vi "Periodic Tasks.vi"() -> ()   [LabVIEW 2011]
doc: "This VI runs in parallel to other tasks. It can contain as many user-defined periodic loops as you need. These can carry out PID or other sorts of timed response."
uses:
  Common/ADXL345 I2C Axis.ctl
  Robot Global Data.vi
panel:
  in  "Driving Sensor Enable":bool=TRUE
  out "Angle":dbl(knob) scale=0.0..360.0
  in  "Reset Zero Position":bool
  out "Robot Angle":dbl
  in  "Inertial Sensors Enable":bool=TRUE
  out "Direction":bool
  out "Voltage Turntable":dbl(knob) scale=160.0..230.0
  out "Acceleration X":dbl
  out "Acceleration Y":dbl
  out "Acceleration Z":dbl
  out "Voltage":dbl(knob) scale=90.0..140.0
  out "Average":dbl
  out "RPM 2":dbl
  out "RPM":dbl(knob) scale=0.0..4000.0
  out "Value":i32
  out "Sonar Distance":dbl
  in  "Shooting Sensor Enable":bool=TRUE
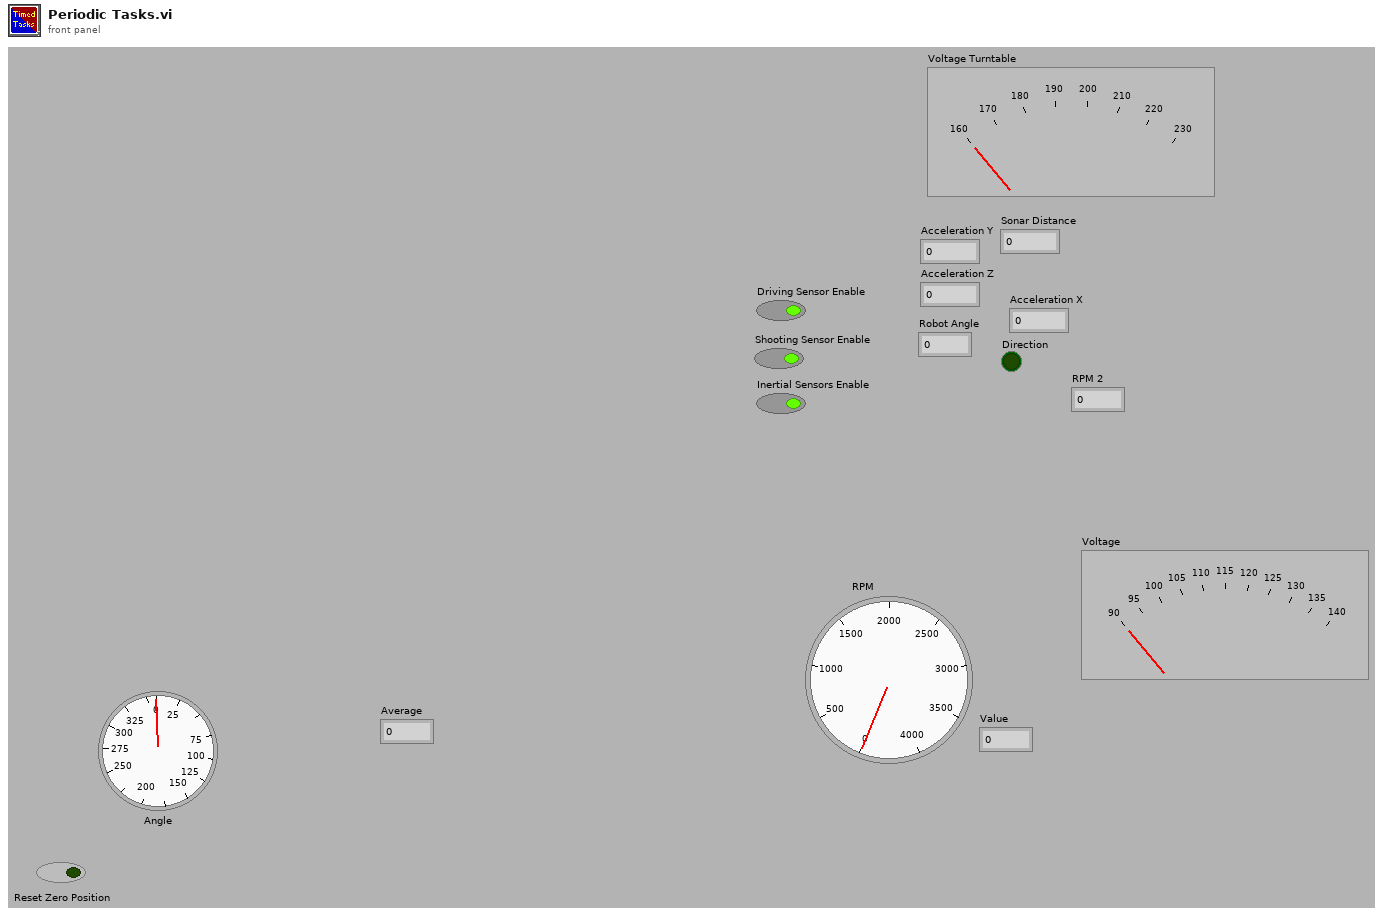
[diagram p1: front panel]
types:
  T1 = typedef "WPI_I2CDevRef.ctl" = cluster{"DevStatus":errorcluster, "Digital Module":T2, "Device Address":u8}
  T2 = typedef "FPGA_TypedefDigitalModule.ctl" = enum16{"Digital Module 1", "Digital Module 2"}
  T3 = typedef "WPI_AnalogChannelDevRef.ctl" = cluster{"DevStatus":errorcluster, "Analog Module":T4, "Analog Channel":T5}
  T4 = typedef "FPGA_TypedefAnalogModule.ctl" = enum16{"Analog Module 1", "Analog Module 2"}
  T5 = typedef "FPGA_AIChannel.ctl" = enum8{"AI 1", "AI 2", "AI 3", "AI 4", "AI 5", "AI 6", "AI 7", "AI 8", "Invalid"}
  T6 = typedef "WPI_CounterDevRef.ctl" = cluster{"DevStatus":errorcluster, "CntIndex":T7}
  T7 = typedef "FPGA_CounterCtrSystemIndex.ctl" = enum8{"Ctr 0", "Ctr 1", "Ctr 2", "Ctr 3", "Ctr 4", "Ctr 5", "Ctr 6", "Ctr 7", "Invalid"}
  T8 = typedef "WPI_GyroDevRef.ctl" = cluster{"DevStatus":errorcluster, "Analog Module":T4, "Analog Channel":T5, "Offset":dbl, "Gain (VoltsPerDegree/Second)":dbl}
  T9 = typedef "WPI_EncoderDevRef.ctl" = cluster{"DevStatus":errorcluster, "EncoderIndex":T10, "CounterIndex":T7, "DistancePerCount":dbl, "Decoding Type":T11}
  T10 = typedef "FPGA_EncoderIdx.ctl" = enum8{"Enc 0", "Enc 1", "Enc 2", "Enc 3", "Invalid"}
  T11 = typedef "WPI_EncoderType.ctl" = enum16{"1x", "2x", "4x"}
  T12 = typedef "ADXL345 I2C Axis.ctl" = u8
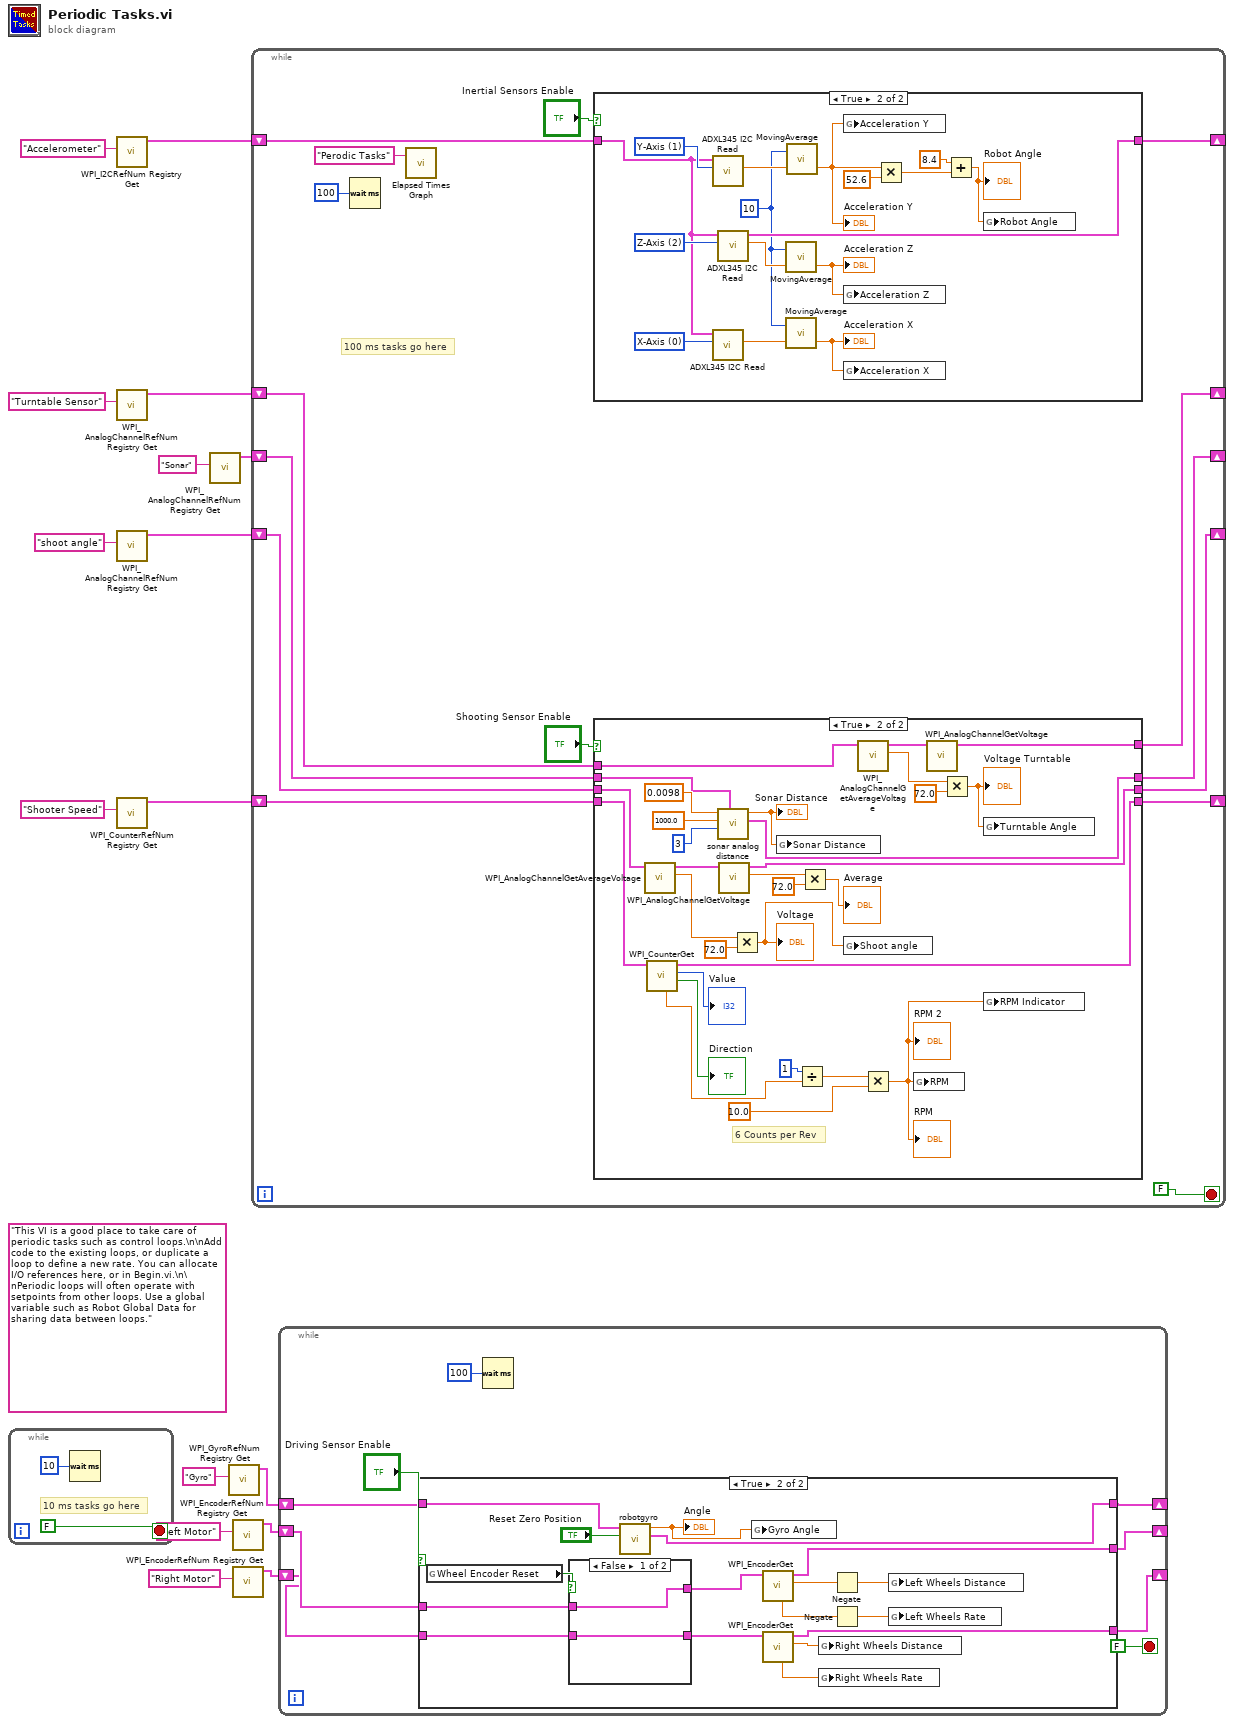
[diagram p0: block diagram]
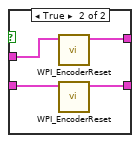
[diagram p3: hidden frame]
diagram:
  (unwired) "This VI is a good place to take care of periodic tasks such as control loops.\n\nAdd code to the existing loops, or duplicate a loop to define a new rate. You can allocate I/O references here, or in Begin.vi.\n\nPeriodic loops will often operate with setpoints from other loops. Use a global variable such as Robot Global Data for sharing data between loops."
  n1 = while {
    stop <- FALSE stop-if-true
    # "10 ms tasks go here"
    n2 = Wait (ms)(milliseconds to wait=u32 10) -> ()  [unwired: 1 out]
  }
  n3 = call <vilib>:"WPI_I2CRefNum Registry Get.vi"("refnum name"="Accelerometer") -> ("I2CDevRef"=w10:T1)  [unwired: 9 in, 1 out]
  n4 = call <vilib>:"WPI_AnalogChannelRefNum Registry Get.vi"("refnum name"="Turntable Sensor") -> ("AIDeviceRef"=w8:T3)  [unwired: 9 in, 1 out]
  n5 = call <vilib>:"WPI_AnalogChannelRefNum Registry Get.vi"("refnum name"="shoot angle") -> ("AIDeviceRef"=w14:T3)  [unwired: 9 in, 1 out]
  n6 = call <vilib>:"WPI_CounterRefNum Registry Get.vi"("refnum name"="Shooter Speed") -> ("CounterDevRef"=w11:T6)  [unwired: 9 in, 1 out]
  n7 = call <vilib>:"WPI_AnalogChannelRefNum Registry Get.vi"("refnum name"="Sonar") -> ("AIDeviceRef"=w16:T3)  [unwired: 9 in, 1 out]
  n8 = call <vilib>:"WPI_GyroRefNum Registry Get.vi"("refnum name"="Gyro") -> ("GyroDevRef"=w1:T8)  [unwired: 9 in, 1 out]
  n9 = call <vilib>:"WPI_EncoderRefNum Registry Get.vi"("refnum name"="Left Motor") -> ("EncoderDevRef"=w4:T9)  [unwired: 9 in, 1 out]
  n10 = call <vilib>:"WPI_EncoderRefNum Registry Get.vi"("refnum name"="Right Motor") -> ("EncoderDevRef"=w3:T9)  [unwired: 9 in, 1 out]
  n11 = while {
    shift-right: [w21] -> _
    shift-left: w10 -> [w20]
    shift-right: [w24] -> _
    shift-left: w8 -> [w23]
    shift-right: [w30] -> _
    shift-left: w14 -> [w31]
    shift-right: [w26] -> _
    shift-left: w16 -> [w27]
    shift-right: [w28] -> _
    shift-left: w11 -> [w29]
    stop <- FALSE stop-if-true
    # "100 ms tasks go here"
    n12 = Wait (ms)(milliseconds to wait=u32 100) -> ()  [unwired: 1 out]
    n13 = call "Elapsed Times Graph.vi"("User Identification:"="Perodic Tasks") -> ()  [unwired: 3 in]
    n14 = case shown="True" "Inertial Sensors Enable" {
      tunnel: [w34 w48] -> w21
      tunnel: w20 -> [w34 w46]
      frame False {
      }
      frame True {
        w40 = 10 ("# to Average")
        w47 = T12 1 items=["X-Axis", "Y-Axis", "Z-Axis"] ("Axis")
        w50 = T12 2 items=["X-Axis", "Y-Axis", "Z-Axis"] ("Axis")
        w49 = T12 0 items=["X-Axis", "Y-Axis", "Z-Axis"] ("Axis")
        n15 = call "ADXL345 I2C Read.vi"("Axis"=w47, "I2CDevRef"=w46) -> ("Acceleration"=w43:dbl)  [unwired: 1 in, 8 out]
        n16 = call "ADXL345 I2C Read.vi"("Axis"=w49, "I2CDevRef"=w46) -> ("Acceleration"=w45:dbl)  [unwired: 1 in, 8 out]
        n17 = call "ADXL345 I2C Read.vi"("Axis"=w50, "I2CDevRef"=w46) -> ("Acceleration"=w42:dbl, "I2CDevRef Out"=w48:T1)  [unwired: 1 in, 7 out]
        n18 = call "MovingAverage.vi"("Additional Value"=w42, "# to Average"=w40) -> ("Moving Average"=w41:dbl)  [unwired: 1 out]
        "Acceleration Z" <- w41
        n19 = call "MovingAverage.vi"("Additional Value"=w45, "# to Average"=w40) -> ("Moving Average"=w44:dbl)  [unwired: 1 out]
        "Acceleration X" <- w44
        n20 = call "MovingAverage.vi"("Additional Value"=w43, "# to Average"=w40) -> ("Moving Average"=w36:dbl)  [unwired: 1 out]
        "Acceleration Y" <- w36
        n21 = global write "Robot Global Data.vi" "Acceleration Y"(w36) -> ()
        n22 = global write "Robot Global Data.vi" "Acceleration Z"(w41) -> ()
        n23 = global write "Robot Global Data.vi" "Acceleration X"(w44) -> ()
        n24 = Multiply(x=w36, y=52.6) -> (x*y=w39:dbl)
        n25 = Add(x=8.4, y=w39) -> (x+y=w35:dbl)
        "Robot Angle" <- w35
        n26 = global write "Robot Global Data.vi" "Robot Angle"(w35) -> ()
      }
    }
    n27 = case shown="True" "Shooting Sensor Enable" {
      tunnel: w31 -> [w52 w77]
      tunnel: [w52 w76] -> w30
      tunnel: w29 -> [w53 w70]
      tunnel: [w53 w69] -> w28
      tunnel: w27 -> [w54 w64]
      tunnel: [w54 w63] -> w26
      tunnel: [w51 w57] -> w24
      tunnel: w23 -> [w51 w58]
      frame False {
      }
      frame True {
        # "6 Counts per Rev"
        n28 = call <vilib>:"WPI_AnalogChannelGetAverageVoltage.vi"("AIDeviceRef"=w77) -> ("Voltage"=w81:dbl, "AIDeviceRef"=w79:T3)  [unwired: 8 in, 1 out]
        n29 = call <vilib>:"WPI_CounterGet.vi"("CounterDevRef in"=w70) -> ("Direction"=→"Direction":bool, "Value"=→"Value":i32, "CounterDevRef out"=w69:T6, "Period (sec)"=w74:dbl)  [unwired: 5 in, 2 out]
        n30 = call "sonar analog distance.vi"("AIDeviceRef in"=w64, "Average Bits"=u8 3, "Samples Per Second"=1000.0, "Scaling factor (V/in)"=0.0098) -> ("AIDeviceRef out"=w63:T3, "distance"=w65:dbl)  [unwired: 5 in, 1 out]
        "Sonar Distance" <- w65
        n31 = call <vilib>:"WPI_AnalogChannelGetVoltage.vi"("AIDeviceRef"=w79) -> ("Voltage"=w78:dbl, "AIDeviceRef"=w76:T3)  [unwired: 8 in, 1 out]
        n32 = Multiply(x=w81, y=72.0) -> (x*y=w84:dbl)
        "Voltage" <- w84
        n33 = global write "Robot Global Data.vi" "Sonar Distance"(w65) -> ()
        n34 = Divide(x=1, y=w74) -> (x/y=w72:dbl)
        n35 = Multiply(x=w78, y=72.0) -> (x*y=→"Average":dbl)
        n36 = global write "Robot Global Data.vi" "Shoot angle"(w84) -> ()
        n37 = call <vilib>:"WPI_AnalogChannelGetAverageVoltage.vi"("AIDeviceRef"=w58) -> ("Voltage"=w60:dbl, "AIDeviceRef"=w61:T3)  [unwired: 8 in, 1 out]
        n38 = Multiply(x=w72, y=10.0) -> (x*y=w62:dbl)
        "RPM 2" <- w62
        "RPM" <- w62
        n39 = global write "Robot Global Data.vi" "RPM"(w62) -> ()
        n40 = call <vilib>:"WPI_AnalogChannelGetVoltage.vi"("AIDeviceRef"=w61) -> ("AIDeviceRef"=w57:T3)  [unwired: 8 in, 2 out]
        n41 = Multiply(x=w60, y=72.0) -> (x*y=w56:dbl)
        "Voltage Turntable" <- w56
        n42 = global write "Robot Global Data.vi" "Turntable Angle"(w56) -> ()
        n43 = global write "Robot Global Data.vi" "RPM Indicator"(w62) -> ()
      }
    }
  }
  n44 = while {
    shift-right: [w90] -> _
    shift-left: w1 -> [w87]
    shift-right: [w89] -> _
    shift-left: w4 -> [w86]
    shift-right: [w88] -> _
    shift-left: w3 -> [w85]
    stop <- FALSE stop-if-true
    n45 = case shown="True" "Driving Sensor Enable" {
      tunnel: w87 -> [w94 w113]
      tunnel: [w94 w110] -> w90
      tunnel: w86 -> [w96 w107]
      tunnel: [w96 w106] -> w89
      tunnel: [w95 w105] -> w88
      tunnel: w85 -> [w95 w104]
      frame False {
      }
      frame True {
        n46 = global read "Robot Global Data.vi" "Wheel Encoder Reset"() -> (w97:bool)
        n47 = case shown="False" w97 {
          tunnel: w107 -> [w115 w119]
          tunnel: w104 -> [w114 w118]
          tunnel: [w114 w117] -> w109
          tunnel: [w115 w116] -> w108
          frame False {
          }
          frame True {
            n48 = call <vilib>:"WPI_EncoderReset.vi"("EncoderDevRef"=w119) -> ("EncoderDevRef"=w116:T9)  [unwired: 9 in, 1 out]
            n49 = call <vilib>:"WPI_EncoderReset.vi"("EncoderDevRef"=w118) -> ("EncoderDevRef"=w117:T9)  [unwired: 9 in, 1 out]
          }
        }
        n50 = call "robotgyro.vi"("Reset Zero Position"="Reset Zero Position", "GyroDevRef in"=w113) -> ("GyroDevRef out"=w110:T8, "Angle"=w111:dbl)  [unwired: 7 in, 1 out]
        "Angle" <- w111
        n51 = global write "Robot Global Data.vi" "Gyro Angle"(w111) -> ()
        n52 = call <vilib>:"WPI_EncoderGet.vi"("EncoderDevRef"=w108) -> ("Distance"=w99:dbl, "EncoderDevRef"=w106:T9, "Rate"=w101:dbl)  [unwired: 5 in, 3 out]
        n53 = call <vilib>:"WPI_EncoderGet.vi"("EncoderDevRef"=w109) -> ("Distance"=w103:dbl, "EncoderDevRef"=w105:T9, "Rate"=w102:dbl)  [unwired: 5 in, 3 out]
        n54 = global write "Robot Global Data.vi" "Right Wheels Distance"(w103) -> ()
        n55 = global write "Robot Global Data.vi" "Right Wheels Rate"(w102) -> ()
        n56 = Negate(x=w99) -> (-x=w98:dbl)
        n57 = Negate(x=w101) -> (-x=w100:dbl)
        n58 = global write "Robot Global Data.vi" "Left Wheels Distance"(w98) -> ()
        n59 = global write "Robot Global Data.vi" "Left Wheels Rate"(w100) -> ()
      }
    }
    n60 = Wait (ms)(milliseconds to wait=u32 100) -> ()  [unwired: 1 out]
  }
